vi "LoadSounds.vi"(8 "error in (no error)":errorcluster, 10 "Path":path, 11 "Game in":refnum<class "Game.lvclass">) -> (0 "error out":errorcluster, 3 "Game out":refnum<class "Game.lvclass">)   [LabVIEW 2019, in "RT_Game.lvlib" / "Game.lvclass"]
uses:
  Game.lvclass
  Game.lvclass/Game.ctl
  <vilib>/rvi/interface/common/niFpgaWaitOnOcc.vi
  <vilib>/Utility/error.llb/Error Cluster From Error Code.vi
  <vilib>/rvi/interface/nirviMethod/nirviMethod.xnode
  FPGA_Interface.ctl
  FPGA Bitfiles/myriogameconsole_FPGATarget_Main_ntsPRcBZGxk.lvbitx
  <vilib>/FPGAPlugInAG/myRIO-1900/niLvFpga_ConfigureFifo_myRIO-1900.vi
  <vilib>/rvi/errors/niLvFpgaMergeErrorWithErrorCode.vi
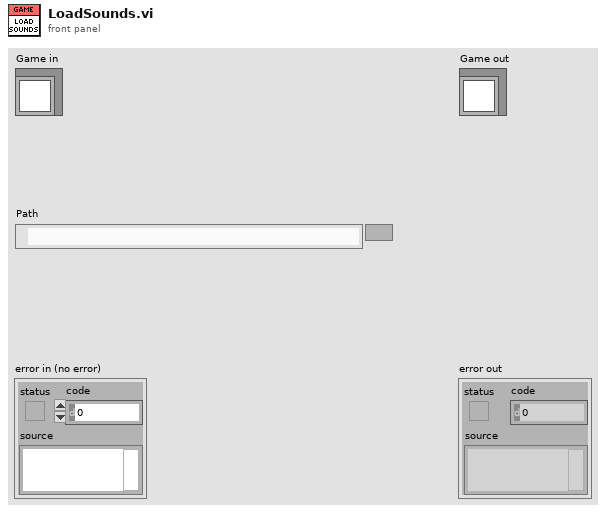
[diagram p1: front panel]
types:
  T1 = typedef "FPGA_Interface.ctl" = refnum<k20>
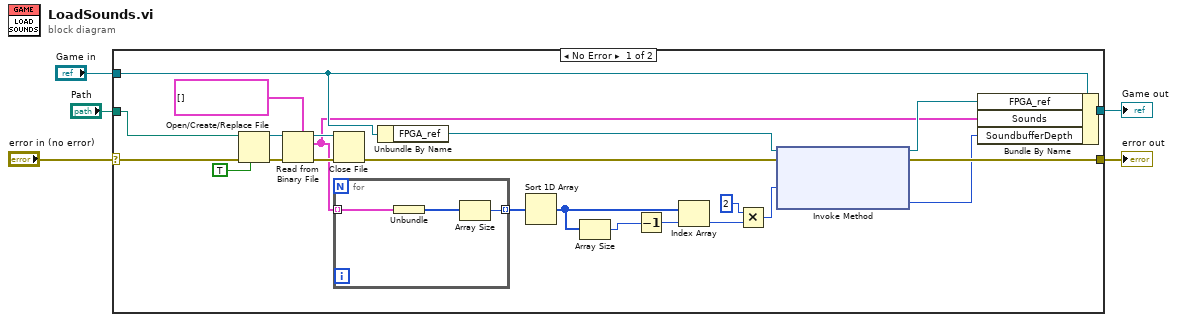
[diagram p0: block diagram]
diagram:
  n1 = case shown="No Error" "error in (no error)" {
    selector: "error in (no error)" -> [w28 w33]
    tunnel: [w19 w33] -> w4
    tunnel: [w22 w32] -> w2
    tunnel: "Game in" -> [w20 w32]
    tunnel: "Path" -> [w21 _]
    frame No Error {
      n2 = Open/Create/Replace File(file path (use dialog)=w21, error in=w28, disable buffering (F)=TRUE) -> (refnum out=w24:refnum<file>, error out=w27:errorcluster)  [unwired: 3 in, 1 out]
      n3 = Read from Binary File(5:cluster{"Sample":i16[]}[] [] ("Samples"), 8:w27, 11:w24) -> (0:w26:errorcluster, 2:w11:cluster{"Sample":i16[]}[], 3:w23:refnum<file>)  [unwired: 3 in, 1 out]
      n4 = Close File(refnum=w23, error in=w26) -> (error out=w25:errorcluster)  [unwired: 1 out]
      n5 = for {
        tunnel: w11 -> [w31] mode=indexing
        tunnel: [w29] -> w10 mode=indexing
        n6 = Unbundle(w31) -> ("Sample"=w30:i16[])
        n7 = Array Size(array=w30) -> (size(s)=w29:i32)
      }
      n8 = Unbundle By Name(w20) -> ("FPGA_ref"=w18:T1)
      n9 = Sort 1D Array(array=w10) -> (sorted array=w8:i32[])
      n10 = Array Size(array=w8) -> (size(s)=w7:i32)
      n11 = Decrement(x=w7) -> (x-1=w6:i32)
      n12 = Index Array(array=w8, index=w6) -> (element=w16:i32)
      n13 = Multiply(x=2, y=w16) -> (x*y=w15:i32)
      n14 = xnode "Invoke Method"("FPGA VI Reference In"=w18, "error in"=w25, "Requested Depth"=w15) -> ("FPGA VI Reference Out"=w17:T1, "error out"=w19:errorcluster, "Actual Depth"=w9:u32)
      n15 = Bundle By Name(cluster=w20, "FPGA_ref"=w17, "Sounds"=w11, "SoundbufferDepth"=w9) -> (w22:refnum<class "Game.lvclass">)
    }
    frame Error {
    }
  }
  "error out" <- w4
  "Game out" <- w2
